vi "iPhone Receive Loop.vi"   [LabVIEW 2014]
uses:
  AccelPacket.ctl
  GyroPacket.ctl
  LocationPacket.ctl
  Global Data.vi
types:
  T1 = typedef "AccelPacket.ctl" = cluster{"Type":u8, "Time":dbl, "Accel X":dbl, "Accel Y":dbl, "Accel Z":dbl}
  T2 = typedef "GyroPacket.ctl" = cluster{"Type":u8, "Time":dbl, "Rotation X":dbl, "Rotation Y":dbl, "Rotation Z":dbl}
  T3 = typedef "LocationPacket.ctl" = cluster{"Type":u8, "Time":dbl, "Lat":dbl, "Long":dbl, "Speed":dbl}
  T4 = cluster{"Accel X":dbl, "Accel Y":dbl, "Accel Z":dbl, "Gyro X":dbl, "Gyro Y":dbl, "Gyro Z":dbl}
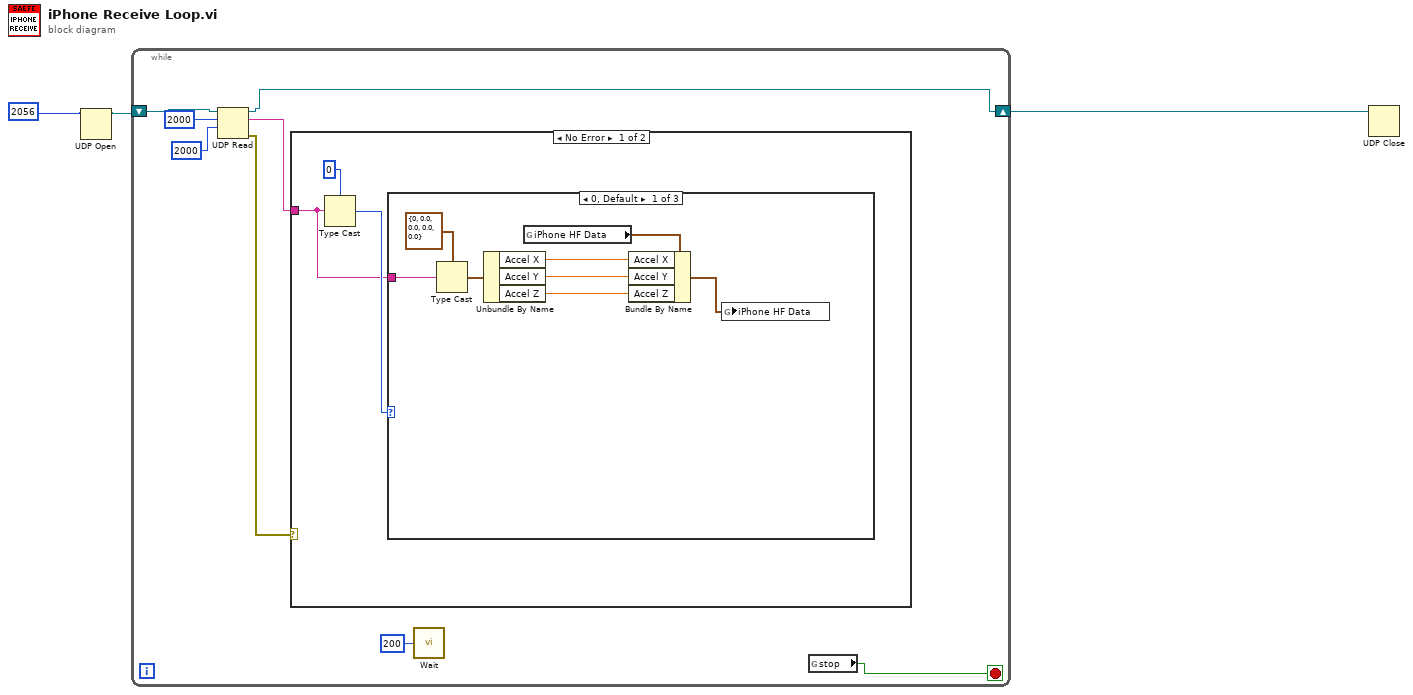
[diagram p0: block diagram]
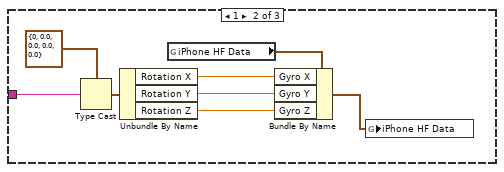
[diagram p2: hidden frame]
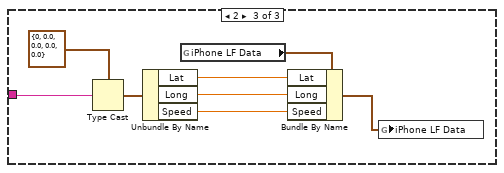
[diagram p3: hidden frame]
diagram:
  n1 = UDP Open(11:u16 2056 ("port")) -> (port=w1:refnum<k16>)  [unwired: 4 in, 2 out]
  n2 = while {
    shift-right: [w10] -> w3
    shift-left: w1 -> [w11]
    stop <- w5 stop-if-true
    n3 = UDP Read(connection ID=w11, max size (548)=2000, timeout ms (25000)=2000) -> (data out=w6:string, error out=w7:errorcluster, 3:w10:refnum<k16>)  [unwired: 1 in, 2 out]
    n4 = case shown="No Error" w7 {
      tunnel: w6 -> [w12 _]
      frame No Error {
        n5 = Type Cast(type=u8 0, x=w12) -> (*(type *) &x=w13:u8)
        n6 = case shown="0, Default" w13 {
          tunnel: w12 -> [w22 w24 w32]
          frame 0, Default {
            n7 = Type Cast(type=T1 {"Type"=0, "Time"=0.0, "Accel X"=0.0, "Accel Y"=0.0, "Accel Z"=0.0} ("AccelPacket"), x=w22) -> (*(type *) &x=w20:T1)
            n8 = Unbundle By Name(w20) -> ("Accel X"=w18:dbl, "Accel Y"=w17:dbl, "Accel Z"=w16:dbl)
            n9 = global read "Global Data.vi" "iPhone HF Data"() -> (w19:T4)
            n10 = Bundle By Name(cluster=w19, "Accel X"=w18, "Accel Y"=w17, "Accel Z"=w16) -> (w15:T4)
            n11 = global write "Global Data.vi" "iPhone HF Data"(w15) -> ()
          }
          frame 1 {
            n12 = Type Cast(type=T2 {"Type"=0, "Time"=0.0, "Rotation X"=0.0, "Rotation Y"=0.0, "Rotation Z"=0.0} ("GyroPacket"), x=w24) -> (*(type *) &x=w30:T2)
            n13 = Unbundle By Name(w30) -> ("Rotation X"=w28:dbl, "Rotation Y"=w27:dbl, "Rotation Z"=w26:dbl)
            n14 = global read "Global Data.vi" "iPhone HF Data"() -> (w29:T4)
            n15 = Bundle By Name(cluster=w29, "Gyro X"=w28, "Gyro Y"=w27, "Gyro Z"=w26) -> (w25:T4)
            n16 = global write "Global Data.vi" "iPhone HF Data"(w25) -> ()
          }
          frame 2 {
            n17 = Type Cast(type=T3 {"Type"=0, "Time"=0.0, "Lat"=0.0, "Long"=0.0, "Speed"=0.0} ("LocationPacket"), x=w32) -> (*(type *) &x=w38:T3)
            n18 = Unbundle By Name(w38) -> ("Lat"=w36:dbl, "Long"=w35:dbl, "Speed"=w34:dbl)
            n19 = global read "Global Data.vi" "iPhone LF Data"() -> (w37:cluster{"Lat":dbl, "Long":dbl, "Speed":dbl})
            n20 = Bundle By Name(cluster=w37, "Lat"=w36, "Long"=w35, "Speed"=w34) -> (w33:cluster{"Lat":dbl, "Long":dbl, "Speed":dbl})
            n21 = global write "Global Data.vi" "iPhone LF Data"(w33) -> ()
          }
        }
      }
      frame Error {
      }
    }
    n22 = call "Wait"("Count(uSec)"=u32 200) -> ()  [unwired: 1 out]
    n23 = global read "Global Data.vi" "stop"() -> (w5:bool)
  }
  n24 = UDP Close(connection ID=w3) -> ()  [unwired: 1 in, 2 out]
